vi "Read XML_001.vi"(8 "error in (no error)":errorcluster, 10 "XML Configuration File Path":path=path "E:/Ballard - Arinc-429 CD/Example Database/Ballard/XML_000.XML", 11 "XML Schema File Path":path=path "E:/Ballard - Arinc-429 CD/Source/System Explorer/SubVIs/Parse XML Ballard/BTI.XSD") -> (0 "error IO":errorcluster, 3 "channels":T1 {"speed" items=["Auto", "Low", "High"]; "Labels"."scheduleBuildUnit" items=["Millisecond", "Microsecond"]})   [LabVIEW 2017]
uses:
  Controls/Ballard_Channel Array.ctl
  Controls/Ballard_Channel.ctl
  Controls/Ballard_Label.ctl
  Controls/Ballard_Word.ctl
  Controls/ARINCParam.ctl
  Shared/Controls and Global/TransferType.ctl
  Controls/Channel_direction.ctl
  Controls/Channel Speed.ctl
  D:/Ballard-Arinc-429-Custom-Device/Source/System Explorer/SubVIs/Parse XML Ballard/Ballard_BTI_XML_Deserializer.dll
  Ballard_BTI_XML_Deserializer.dll
  Ballard Arinc-429 System Explorer.lvlib
  Shared/Ballard Arinc-429 Shared.lvlib
panel:
  out "name":string
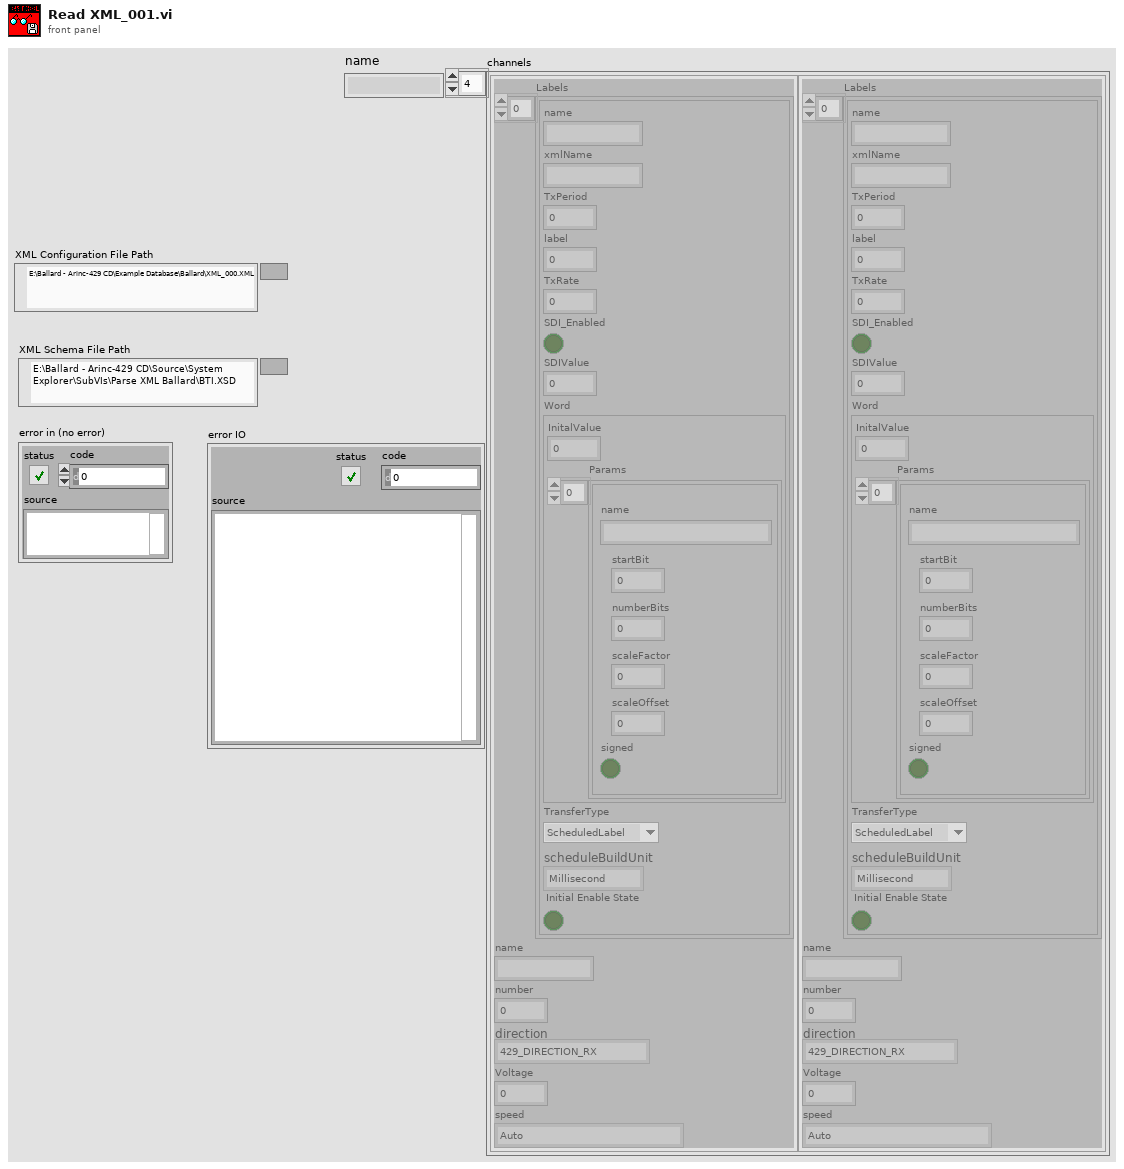
[diagram p1: front panel]
types:
  T1 = typedef "Ballard Arinc-429 System Explorer.lvlib/Ballard_Channel Array.ctl" = T2[]
  T2 = typedef "Ballard Arinc-429 System Explorer.lvlib/Ballard_Channel.ctl" = cluster{"Labels":T3[], "name":string, "number":u8, "direction":T7, "Voltage":dbl, "speed":T8}
  T3 = typedef "Ballard Arinc-429 System Explorer.lvlib/Ballard_Label.ctl" = cluster{"name":string, "xmlName":string, "TxPeriod":u32, "label":u32, "TxRate":dbl, "SDI_Enabled":bool, "SDIValue":u8, "Word":T4, "TransferType":T6, "scheduleBuildUnit":i32, "Initial Enable State":bool}
  T4 = typedef "Ballard Arinc-429 System Explorer.lvlib/Ballard_Word.ctl" = cluster{"InitalValue":u32, "Params":T5[]}
  T5 = typedef "Ballard Arinc-429 System Explorer.lvlib/ARINCParam.ctl" = cluster{"name":string, "startBit":i32, "numberBits":i32, "scaleFactor":dbl, "scaleOffset":dbl, "signed":bool}
  T6 = typedef "Ballard Arinc-429 Shared.lvlib/TransferType.ctl" = enum16{"ScheduledLabel", "Acyclic", "Block", "Strobe"}
  T7 = typedef "Ballard Arinc-429 System Explorer.lvlib/Channel_direction.ctl" = enum16{"429_DIRECTION_RX", "429_DIRECTION_TX"}
  T8 = typedef "Ballard Arinc-429 System Explorer.lvlib/Channel Speed.ctl" = i32
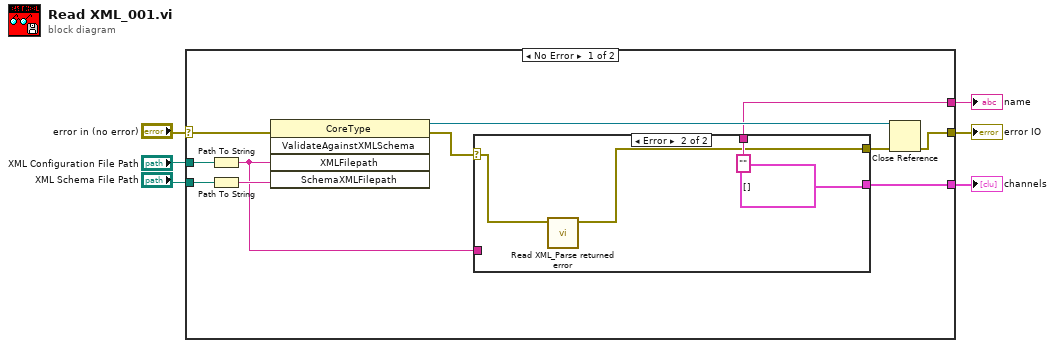
[diagram p0: block diagram]
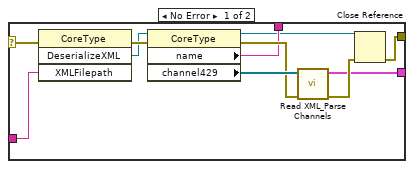
[diagram p2: hidden frame]
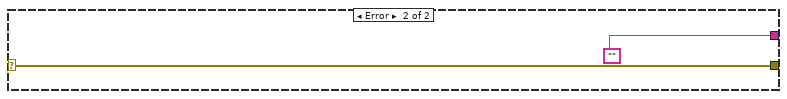
[diagram p3: hidden frame]
diagram:
  n1 = case shown="No Error" "error in (no error)" {
    selector: "error in (no error)" -> [w9 w34]
    tunnel: "XML Configuration File Path" -> [w17 _]
    tunnel: "XML Schema File Path" -> [w16 _]
    tunnel: [w13 w34] -> w3
    tunnel: [w11 _] -> w2
    tunnel: [w10 "" ("name")] -> w1
    frame No Error {
      n2 = Path To String(path=w17) -> (string=w8:string)
      n3 = Path To String(path=w16) -> (string=w15:string)
      n4 = invoke class="CoreType" method="ValidateAgainstXMLSchema"(error in=w9, "XMLFilepath"=w8, "SchemaXMLFilepath"=w15) -> (reference out=w12:refnum<k24>, error out=w7:errorcluster)  [unwired: 2 in, 3 out]
      n5 = case shown="Error" w7 {
        selector: w7 -> [w18 w30]
        tunnel: [w25 w29] -> w14
        tunnel: [w24 T2[] [] ("Array")] -> w11
        tunnel: [w23 "" ("name")] -> w10
        tunnel: w8 -> [w21 _]
        frame No Error {
          n6 = invoke class="CoreType" method="DeserializeXML"(error in=w18, "XMLFilepath"=w21) -> (error out=w20:errorcluster, "DeserializeXML"=w19:refnum<k24>)  [unwired: 2 in, 2 out]
          n7 = property class="CoreType"(reference=w19, error in=w20) -> (reference out=w22:refnum<k24>, error out=w27:errorcluster, "name"=w23:string, "channel429"=w28:refnum<k24>[])
          n8 = call "Read XML_Parse Channels.vi"("error in (no error)"=w27, "channel429"=w28) -> ("error out"=w26:errorcluster, "Array"=w24:T2[])  [unwired: 8 in]
          n9 = Close Reference(reference=w22, error in (no error)=w26) -> (error out=w25:errorcluster)
        }
        frame Error {
          n10 = call "Read XML_Parse returned error.vi"("error in (no error)"=w30) -> ("error out"=w29:errorcluster)  [unwired: 10 in]
        }
      }
      n11 = Close Reference(reference=w12, error in (no error)=w14) -> (error out=w13:errorcluster)
    }
    frame Error {
    }
  }
  "channels" <- w2
  "error IO" <- w3
  "name" <- w1
